vi "ReorderRGB.vi"(1 "pImage in":u16[](array[numeric])) -> (0 "pImage out":u16[](array[numeric]))   [LabVIEW 2013, in "VRI.lvlib"]
uses:
  VRI.lvlib
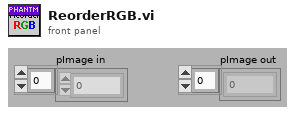
[diagram p1: front panel]
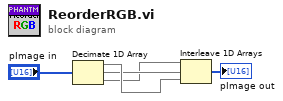
[diagram p0: block diagram]
diagram:
  n1 = Decimate 1D Array("pImage in") -> (w4:u16[], w3:u16[], w2:u16[])
  n2 = Interleave 1D Arrays(w2, w3, w4) -> (→"pImage out":u16[])
